vi "Find Moves.vi"(7 "Part 1":bool, 8 "error in (no error)":errorcluster, 9 "Remaining Excursions":cluster{"A":u8, "B":u8, "C":u8, "D":u8}, 10 "Amphipods in":refnum<class "Amphipod.lvclass">[](array[class]), 11 "Amphipod in":refnum<class "Amphipod.lvclass">) -> (0 "error out":errorcluster, 1 "Remaining Excursions for Moves":cluster{"A":u8, "B":u8, "C":u8, "D":u8}[](array[cluster]), 2 "Valid Moves":cluster{"Row":i8, "Column":i8}[](array[cluster]), 3 "Amphipod out":refnum<class "Amphipod.lvclass">)   [LabVIEW 2019, in "23.lvlib" / "Amphipod.lvclass"]
uses:
  Amphipod.lvclass
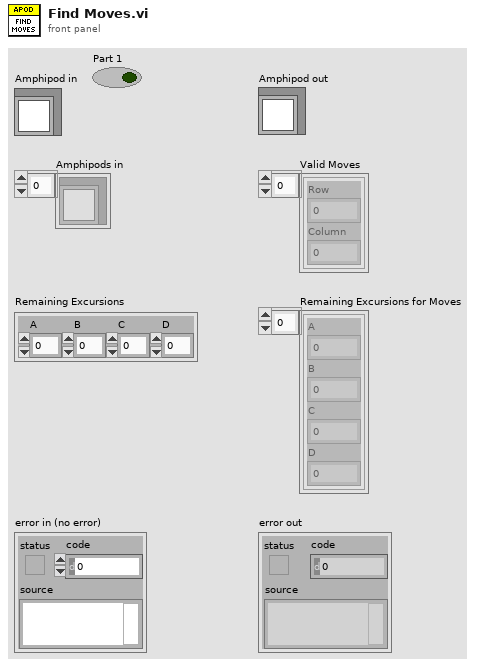
[diagram p1: front panel]
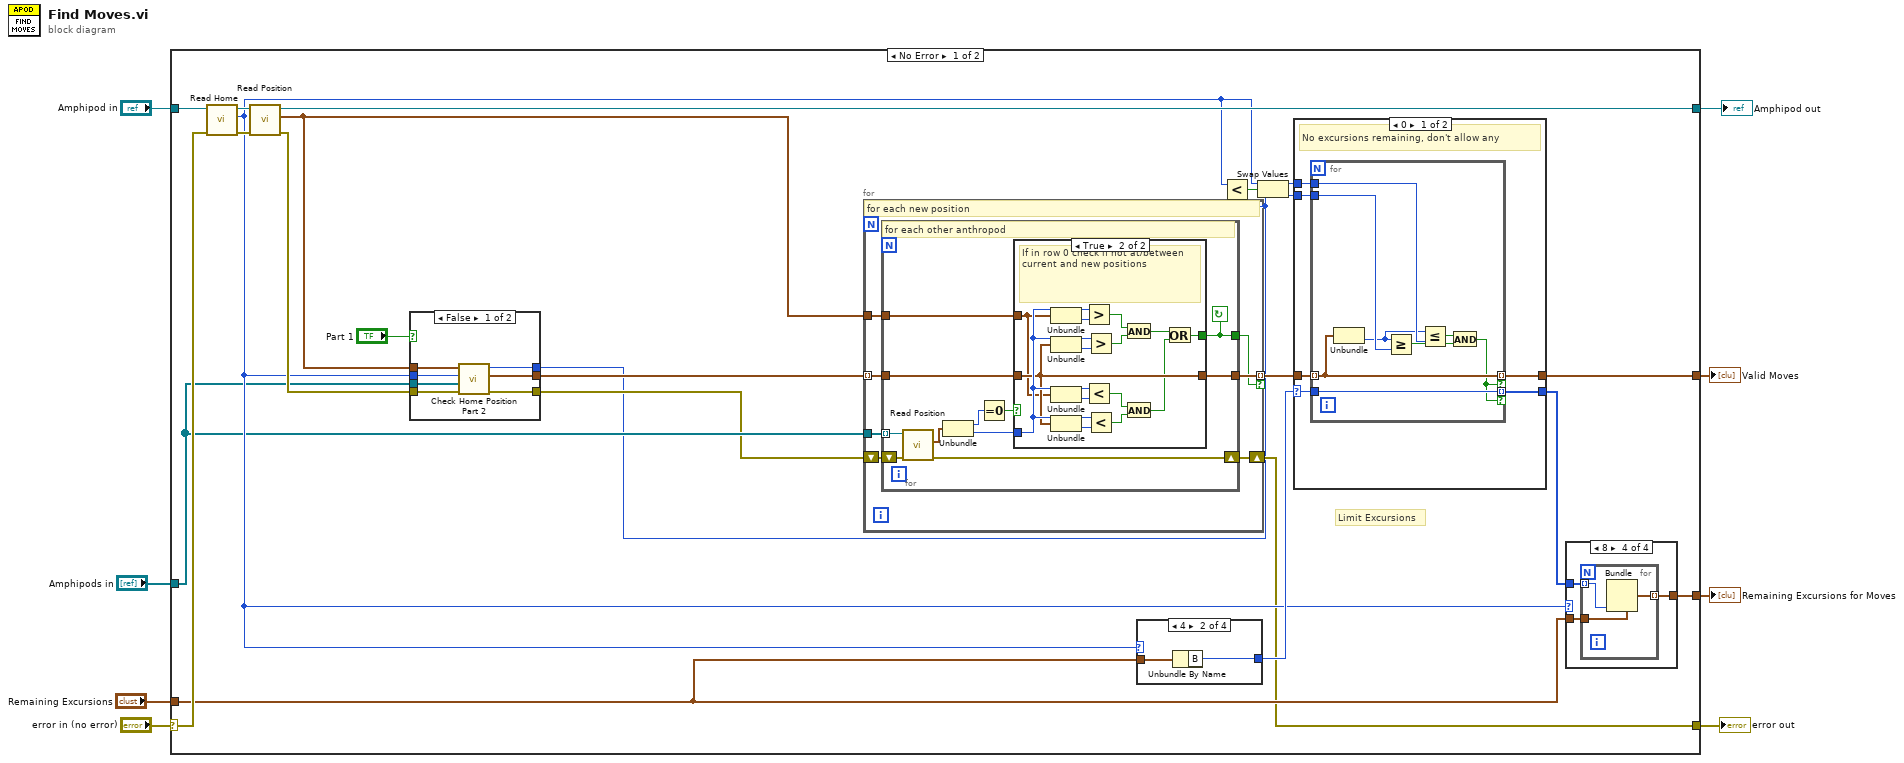
[diagram p0: block diagram]
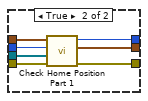
[diagram p2: hidden frame]
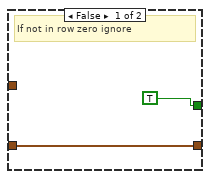
[diagram p3: hidden frame]
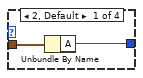
[diagram p4: hidden frame]
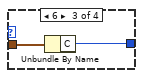
[diagram p5: hidden frame]
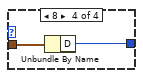
[diagram p6: hidden frame]
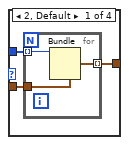
[diagram p7: hidden frame]
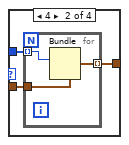
[diagram p8: hidden frame]
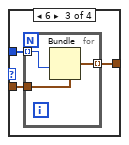
[diagram p9: hidden frame]
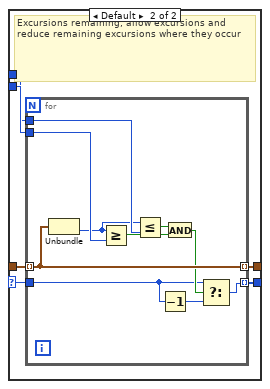
[diagram p10: hidden frame]
diagram:
  n1 = case shown="No Error" "error in (no error)" {
    selector: "error in (no error)" -> [w28 w143]
    tunnel: [w11 w143] -> w7
    tunnel: "Amphipod in" -> [w29 w142]
    tunnel: "Amphipods in" -> [w15 _]
    tunnel: [w31 w142] -> w4
    tunnel: [w18 _] -> w2
    tunnel: "Remaining Excursions" -> [w21 _]
    tunnel: [w19 _] -> w1
    frame No Error {
      # "Limit Excursions"
      n2 = call-dynamic "Read Home.vi"("error in (no error)"=w28, "Amphipod in"=w29) -> ("error out"=w27:errorcluster, "Home"=w17:i8, "Amphipod out"=w30:refnum<class "Amphipod.lvclass">)  [unwired: 7 in]
      n3 = call-dynamic "Read Position.vi"("error in (no error)"=w27, "Amphipod in"=w30) -> ("error out"=w26:errorcluster, "Position"=w14:cluster{"Row":i8, "Column":i8}, "Amphipod out"=w31:refnum<class "Amphipod.lvclass">)  [unwired: 7 in]
      n4 = case shown="False" "Part 1" {
        tunnel: w26 -> [w35 w45]
        tunnel: w17 -> [w37 w44]
        tunnel: [w33 w43] -> w16
        tunnel: w15 -> [w36 w42]
        tunnel: w14 -> [w38 w41]
        tunnel: [w34 w40] -> w13
        tunnel: [w32 w39] -> w10
        frame False {
          n5 = call "Check Home Position Part 2.vi"("error in (no error)"=w35, "Amphipods in"=w36, "Home"=w37, "Position in"=w38) -> ("error out"=w34:errorcluster, "Position out"=w33:cluster{"Row":i8, "Column":i8}[], "Column"=w32:i8)  [unwired: 5 in]
        }
        frame True {
          n6 = call "Check Home Position Part 1.vi"("error in (no error)"=w45, "Amphipods in"=w42, "Home"=w44, "Position in"=w41) -> ("error out"=w40:errorcluster, "Position out"=w43:cluster{"Row":i8, "Column":i8}[], "Column"=w39:i8)  [unwired: 5 in]
        }
      }
      n7 = for {
        tunnel: w16 -> [w51] mode=indexing
        tunnel: w15 -> [w52]
        tunnel: w14 -> [w50]
        shift-right: [w48] -> w11
        shift-left: w13 -> [w49]
        tunnel: [w47] -> w12 mode=indexing if=w46
        # "for each new position"
        n8 = for {
          tunnel: w52 -> [w63] mode=indexing
          tunnel: w51 -> [w55]
          tunnel: w50 -> [w62]
          shift-right: [w58] -> w48
          shift-left: w49 -> [w59]
          tunnel: [w54] -> w47
          tunnel: [w53] -> w46
          stop <- w53 continue-if-true
          # "for each other anthropod"
          n9 = call-dynamic "Read Position.vi"("error in (no error)"=w59, "Amphipod in"=w63) -> ("error out"=w58:errorcluster, "Position"=w61:cluster{"Row":i8, "Column":i8})  [unwired: 7 in, 1 out]
          n10 = Unbundle(w61) -> ("Row"=w60:i8, "Column"=w57:i8)
          n11 = Equal To 0?(x=w60) -> (x = 0?=w56:bool)
          n12 = case shown="True" w56 {
            tunnel: w62 -> [_ w69]
            tunnel: w55 -> [w65 w70]
            tunnel: w57 -> [_ w71]
            tunnel: [w65 w70] -> w54
            tunnel: [TRUE w66] -> w53
            frame False {
              # "If not in row zero ignore"
            }
            frame True {
              # "If in row 0 check if not at/between current and new positions"
              n13 = Unbundle(w69) -> ("Column"=w79:i8)  [unwired: 1 out]
              n14 = Unbundle(w70) -> ("Column"=w78:i8)  [unwired: 1 out]
              n15 = Unbundle(w69) -> ("Column"=w72:i8)  [unwired: 1 out]
              n16 = Unbundle(w70) -> ("Column"=w73:i8)  [unwired: 1 out]
              n17 = Greater?(x=w71, y=w79) -> (0:w77:bool)
              n18 = Less?(x=w71, y=w72) -> (x < y?=w74:bool)
              n19 = Greater?(x=w71, y=w78) -> (0:w76:bool)
              n20 = Less?(x=w71, y=w73) -> (x < y?=w75:bool)
              n21 = And(x=w77, y=w76) -> (x .and. y?=w67:bool)
              n22 = And(x=w74, y=w75) -> (x .and. y?=w68:bool)
              n23 = Or(x=w67, y=w68) -> (x .or. y?=w66:bool)
            }
          }
        }
      }
      n24 = case shown="4" w17 {
        tunnel: w21 -> [w81 w83 w85 w87]
        tunnel: [w80 w82 w84 w86] -> w23
        frame 2, Default {
          n25 = Unbundle By Name(w81) -> ("A"=w80:u8)
        }
        frame 4 {
          n26 = Unbundle By Name(w83) -> ("B"=w82:u8)
        }
        frame 6 {
          n27 = Unbundle By Name(w85) -> ("C"=w84:u8)
        }
        frame 8 {
          n28 = Unbundle By Name(w87) -> ("D"=w86:u8)
        }
      }
      n29 = Less?(x=w17, y=w10) -> (x < y?=w25:bool)
      n30 = Swap Values(12:w17, 13:w25, 14:w10) -> (1:w22:i8, 3:w24:i8)
      n31 = case shown="0" w23 {
        selector: w23 -> [w113 w127]
        tunnel: w12 -> [w117 w131]
        tunnel: [w116 w130] -> w18
        tunnel: w24 -> [w115 w129]
        tunnel: w22 -> [w114 w128]
        tunnel: [w112 w126] -> w20
        frame 0 {
          # "No excursions remaining, don't allow any"
          n32 = for {
            tunnel: w117 -> [w125] mode=indexing
            tunnel: [w125] -> w116 mode=indexing if=w119
            tunnel: w115 -> [w124]
            tunnel: w114 -> [w123]
            tunnel: w113 -> [w120]
            tunnel: [w120] -> w112 mode=indexing if=w119
            n33 = Unbundle(w125) -> ("Column"=w118:i8)  [unwired: 1 out]
            n34 = Greater Or Equal?(x=w118, y=w124) -> (x >= y?=w121:bool)
            n35 = Less Or Equal?(x=w118, y=w123) -> (x <= y?=w122:bool)
            n36 = And(x=w122, y=w121) -> (x .and. y?=w119:bool)
          }
        }
        frame Default {
          # "Excursions remaining, allow excursions and reduce remaining excursions where they occur"
          n37 = for {
            tunnel: w131 -> [w141] mode=indexing
            tunnel: [w141] -> w130 mode=indexing
            tunnel: w129 -> [w140]
            tunnel: w128 -> [w139]
            tunnel: w127 -> [w133]
            tunnel: [w135] -> w126 mode=indexing
            n38 = Unbundle(w141) -> ("Column"=w132:i8)  [unwired: 1 out]
            n39 = Greater Or Equal?(x=w132, y=w140) -> (x >= y?=w137:bool)
            n40 = Less Or Equal?(x=w132, y=w139) -> (x <= y?=w138:bool)
            n41 = Decrement(x=w133) -> (x-1=w134:u8)
            n42 = And(x=w138, y=w137) -> (x .and. y?=w136:bool)
            n43 = Select(t=w133, s=w136, f=w134) -> (s? t:f=w135:u8)
          }
        }
      }
      n44 = case shown="8" w17 {
        tunnel: w21 -> [w90 w96 w102 w108]
        tunnel: [w88 w94 w100 w106] -> w19
        tunnel: w20 -> [w89 w95 w101 w107]
        frame 2, Default {
          n45 = for {
            tunnel: w90 -> [w93]
            tunnel: w89 -> [w92] mode=indexing
            tunnel: [w91] -> w88 mode=indexing
            n46 = Bundle(cluster=w93, "A"=w92) -> (w91:cluster{"A":u8, "B":u8, "C":u8, "D":u8})  [unwired: 3 in]
          }
        }
        frame 4 {
          n47 = for {
            tunnel: w96 -> [w99]
            tunnel: w95 -> [w97] mode=indexing
            tunnel: [w98] -> w94 mode=indexing
            n48 = Bundle(cluster=w99, "B"=w97) -> (w98:cluster{"A":u8, "B":u8, "C":u8, "D":u8})  [unwired: 3 in]
          }
        }
        frame 6 {
          n49 = for {
            tunnel: w102 -> [w105]
            tunnel: w101 -> [w103] mode=indexing
            tunnel: [w104] -> w100 mode=indexing
            n50 = Bundle(cluster=w105, "C"=w103) -> (w104:cluster{"A":u8, "B":u8, "C":u8, "D":u8})  [unwired: 3 in]
          }
        }
        frame 8 {
          n51 = for {
            tunnel: w108 -> [w111]
            tunnel: w107 -> [w109] mode=indexing
            tunnel: [w110] -> w106 mode=indexing
            n52 = Bundle(cluster=w111, "D"=w109) -> (w110:cluster{"A":u8, "B":u8, "C":u8, "D":u8})  [unwired: 3 in]
          }
        }
      }
    }
    frame Error {
    }
  }
  "error out" <- w7
  "Amphipod out" <- w4
  "Valid Moves" <- w2
  "Remaining Excursions for Moves" <- w1
